vi "Seq Station Part Config.vi"(6 "User Name":string="Jon", 8 "Level":i32, 10 "station default states":T1[](array[typedef]) {"LIN INFO"."NAD" format="%.0x"; "LIN INFO"."ADCS LIN"."HW select" items=["NI-XNET", "NI-CAN"]; "LVDT Status"."LVDT's stored config"."Lower Limit" format="%.2f"; "LVDT Status"."LVDT's stored config"."Upper Limit" format="%.2f"; "Store Data"."Sun Shade Open Force Limits"."Variance" format="%.2g"; "Store Data"."Sun Shade Open Force Limits"."Truncation End" format="%.2g"; "Store Data"."Sun Shade Open Force Limits"."Truncation Start" format="%.2g"; "Store Data"."Sun Shade Open Force Limits"."Avg Max" format="%.2g"; "Store Data"."Sun Shade Open Force Limits"."Avg Min" format="%.2g"; "Store Data"."Sun Shade Open Force Limits"."Overall Max" format="%.2g"; "Store Data"."Sun Shade Open Force Limits"."Overall Min" format="%.2g"; "Store Data"."Sun Shade Close Force Limits"."Variance" format="%.2g"; "Store Data"."Sun Shade Close Force Limits"."Truncation End" format="%.2g"; "Store Data"."Sun Shade Close Force Limits"."Truncation Start" format="%.2g"; "Store Data"."Sun Shade Close Force Limits"."Avg Max" format="%.2g"; "Store Data"."Sun Shade Close Force Limits"."Avg Min" format="%.2g"; "Store Data"."Sun Shade Close Force Limits"."Overall Max" format="%.2g"; "Store Data"."Sun Shade Close Force Limits"."Overall Min" format="%.2g"; "Store Data"."Motion Data Array"."Motion Data Limits"."LIN Msg"."Msg" format="%02x"; "Store Data"."Motion Data Array"."Motion Data Limits"."LIN Msg"."ID" format="%02x"}, 11 "Base Path":path=path "C:/Labview Code") -> ()   [LabVIEW 2018]
uses:
  02.Type Def's/main state cluster.ctl
  02.Type Def's/All Switch Configuration Cluster.ctl
  02.Type Def's/All Motions.ctl
  02.Type Def's/EOL Switch Value Configuration Cluster.ctl
  02.Type Def's/EOL Switch Max Min Check Cluster.ctl
  02.Type Def's/station nvh config.ctl
  02.Type Def's/station rs232 port map.ctl
  02.Type Def's/station ethernet address map.ctl
  02.Type Def's/station paths.ctl
  02.Type Def's/EOL Save Module Test Data Control.ctl
  02.Type Def's/EOL Motion Database Table.ctl
  05.UserVI's/type defs/17x Audit Motion Data Seq Control.ctl
  05.UserVI's/type defs/17x AP Data Type.ctl
  05.UserVI's/type defs/17x Sunshade Limts Seq.ctl
  02.Type Def's/EOL Module Info Control.ctl
  02.Type Def's/station DI map.ctl
  05.UserVI's/type defs/EOL Global Digital Input Control.ctl
  02.Type Def's/control refs.ctl
  02.Type Def's/station motion data indicator.ctl
  02.Type Def's/Screen Motion Data.ctl
  02.Type Def's/Pass Fail Control.ctl
  02.Type Def's/station hmi.ctl
  02.Type Def's/lvdt name val pair.ctl
  02.Type Def's/individual station status.ctl
  02.Type Def's/misc station config.ctl
  05.UserVI's/Lambda Power/power supply types.ctl
  05.UserVI's/type defs/EOL LVDT's Check Controller.ctl
  05.UserVI's/LVDT's/lvdt precision.ctl
  02.Type Def's/sequence state.ctl
  05.UserVI's/sequence/type defs/Sequence Info.ctl
  05.UserVI's/type defs/EOL Part Setup.ctl
  02.Type Def's/All Communication Types.ctl
  05.UserVI's/type defs/Communication with Motors.ctl
  05.UserVI's/type defs/RAP Signal Control.ctl
  05.UserVI's/type defs/EOL Motor Type.ctl
  02.Type Def's/station LIN config.ctl
  03.Inalfa LIN/LIN Device.ctl
  <vilib>/CMC.AME/Inalfa ADCS/Ctl'Def/ADCS_LIN info.ctl
  C:/Program Files (x86)/National Instruments/LabVIEW 2018/vi.lib/CMC.AME/Inalfa TS LIN/TOSUN/TSMaster/bin/Interop.TSMasterAPI.dll
  Program Files (x86)/National Instruments/LabVIEW 2018/vi.lib/CMC.AME/Inalfa TS LIN/TOSUN/TSMaster/bin/Interop.TSMasterAPI.dll
  06.Test Loop/Sub'VIs/Type Def's/Config Info.ctl
panel:
  in  "LIN Msg Editor":bool
  in  "st4":bool
  in  "st3":bool
  in  "shade config":bool
  in  "st0":bool
  in  "Part Type":u16(ring) items=["OE", "EX1H", "EX1E"]
  in  "st1":bool
  in  "Exit":bool
  in  "st2":bool
  # "Part Configuration"
  # "Sunroof Barcode"
  # "Pallet Number"
  # "Part Type"
  # "Application Status"
  # "Current Step"
  # "Cycle Time"
  # "Pass / Fail"
  # "Shade Close"
  # "Actual Data"
  # "Limits"
  # "Avg Current"
  # "Run Time"
  # "Speed"
  # "Noise Test"
  # "Position"
  # "Shade Open"
  # "Actual Data"
  # "Limits"
  # "Avg Current"
  # "Run Time"
  # "Speed"
  # "Noise Test"
  # "Position"
  # "Vent Close"
  # "Actual Data"
  # "Limits"
  # "Avg Current"
  # "Run Time"
  # "Speed"
  # "Noise Test"
  # "Position"
  # "Vent Open"
  # "Actual Data"
  # "Limits"
  # "Avg Current"
  # "Run Time"
  # "Speed"
  # "Noise Test"
  # "Position"
  # "Slide Close"
  # "Actual Data"
  # "Limits"
  # "Avg Current"
  # "Run Time"
  # "Speed"
  # "Noise Test"
  # "Position"
  # "Slide Open"
  # "Actual Data"
  # "Limits"
  # "Avg Current"
  # "Run Time"
  # "Speed"
  # "Noise Test"
  # "Position"
  # "Min"
  # "N"
  # "Min"
  # "Start"
  # "N"
  # "Max"
  # "N"
  # "Max"
  # "N"
  # "End"
  # "Min"
  # "N"
  # "Min"
  # "Start"
  # "N"
  # "Max"
  # "N"
  # "Max"
  # "N"
  # "End"
  # "Min"
  # "Max"
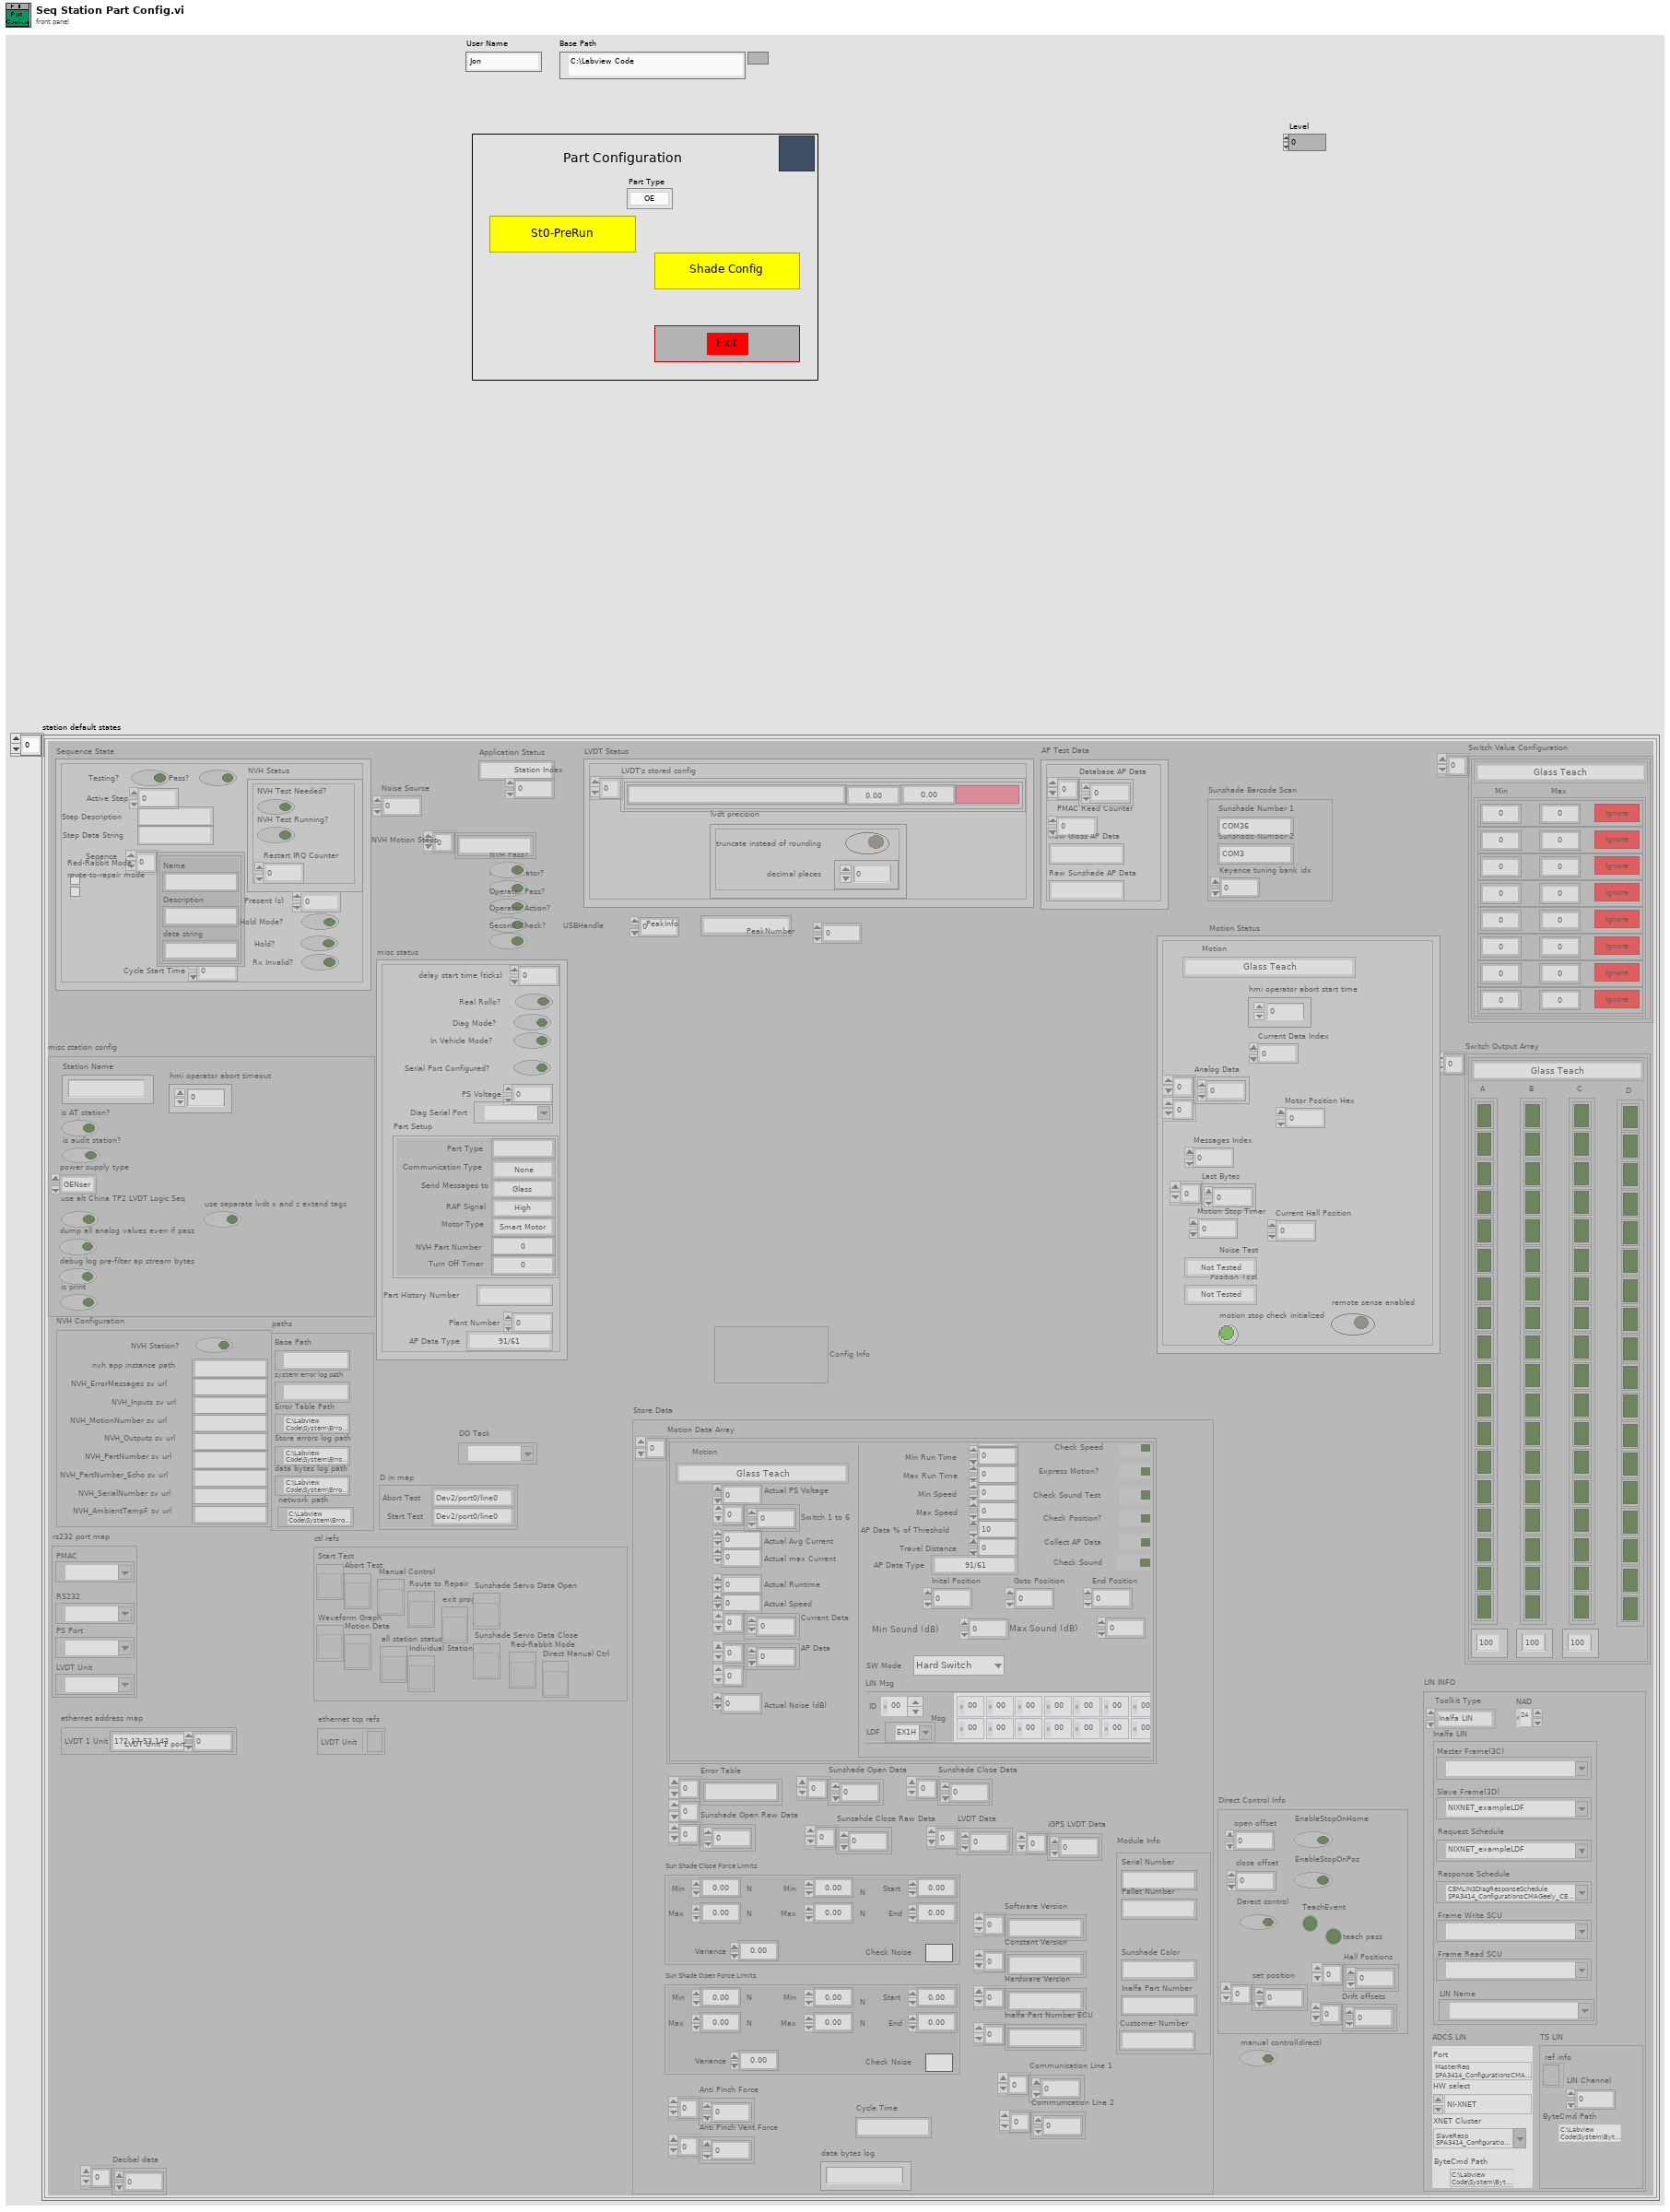
[diagram p1: front panel]
types:
  T1 = typedef "main state cluster.ctl" = cluster{"Application Status":string, "Switch Output Array":T2[], "Switch Value Configuration":T4[], "NVH Configuration":T6, "rs232 port map":T7, "ethernet address map":T8, "paths":T9, "Station Index":i32, "Store Data":T10, "D in map":T16, "DO Task":refnum<k21>, "ctl refs":T18, "misc station config":T19, "ethernet tcp refs":cluster{"LVDT Unit":refnum<k5>}, "Sunshade Barcode Scan":cluster{"Sunshade Number 2":string, "Sunshade Number 1":string, "Keyence tuning bank idx":i32}, "AP Test Data":cluster{"Raw Sunshade AP Data":string, "Raw Glass AP Data":string, "PMAC Read Counter":dbl, "Database AP Data":dbl[]}, "Motion Status":cluster{"hmi operator abort start time":u32, "Current Data Index":i32, "Analog Data":sgl[][], "Motor Position Hex":u16, "Messages Index":u16, "Last Bytes":u8[], "Current Hall Position":i16, "Motion Stop Timer":u32, "Position Test":T21, "Noise Test":T21, "motion stop check initialized":bool, "remote sense enabled":bool, "Motion":T3}, "LVDT Status":cluster{"LVDT's stored config":T22[], "lvdt precision":T23}, "Sequence State":T24, "misc status":cluster{"delay start time (ticks)":u32, "In Vehicle Mode?":bool, "Diag Mode?":bool, "Serial Port Configured?":bool, "PS Voltage":dbl, "Diag Serial Port":refnum<visa-resource-name>, "Part Setup":T26, "Part History Number":string, "Plant Number":u8, "AP Data Type":T13, "Real Rollo?":bool}, "NVH Operator?":bool, "NVH Pass?":bool, "Operator Pass?":bool, "Operator Action?":bool, "Noise Source":u32, "USBHandle":i32, "PeakInfo":string, "PeakNumber":i32, "NVH Motion Steps":string[], "Second Check?":bool, "Decibel data":dbl[], "Direct Control Info":cluster{"EnableStopOnHome":bool, "EnableStopOnPos":bool, "TeachEvent":bool, "open offset":i32, "close offset":i32, "Derect control":bool, "set position":i32[], "teach pass ":bool, "Drift offsets":i32[], "Hall Positions":i32[]}, "manual control(direct)":bool, "LIN INFO":T31, "Config Info":T34}
  T2 = typedef "All Switch Configuration Cluster.ctl" = cluster{"All Motions":T3, "A":bool[], "B":bool[], "C":bool[], "D":bool[], "A activation time (ms)":u32, "B activation time (ms)":u32, "C activation time (ms)":u32}
  T3 = typedef "All Motions.ctl" = enum16{"Glass Teach", "Glass Slide Open", "Glass Slide Close", "Glass Vent Open", "Glass Vent Close", "Sunshade Teach", "Sunshade Open", "Sunshade Close", "Idle", "Sunshade Open 2", "Sunshade Close 2", "Glass Slide Open Sunshade Open", "Glass Slide Open Sunshade Close", "Glass Slide Close Sunshade Open", "Glass Slide Close Sunshade Close", "Glass Vent Open Sunshade Open", "Glass Vent Open Sunshade Close", "Glass Vent Close Sunshade Open", "Glass Vent Close Sunshade Close", "Express Glass Slide Open", "Express Glass Slide Close", "Express Glass Vent Open", "Express Glass Vent Close", "Express Sunshade Open", "Express Sunshade Close", "Express Sunshade Open 2", "Express Sunshade Close 2", "Express Glass Slide Open Sunshade Open", "Express Glass Slide Open Sunshade Close", "Express Glass Slide Close Sunshade Open", "Express Glass Slide Close Sunshade Close", "Express Glass Vent Open Sunshade Open", "Express Glass Vent Open Sunshade Close", "Express Glass Vent Close Sunshade Open", "Express Glass Vent Close Sunshade Close", "Goto Position Glass", "Goto Position Sunshade", "Sunshade Teach 2"}
  T4 = typedef "EOL Switch Value Configuration Cluster.ctl" = cluster{"All Motions":T3, "Array":T5[]}
  T5 = typedef "EOL Switch Max Min Check Cluster.ctl" = cluster{"Min":dbl, "Max":dbl, "Check?":bool}
  T6 = typedef "station nvh config.ctl" = cluster{"NVH Station?":bool, "nvh app instance path":string, "NVH_ErrorMessages sv url":string, "NVH_Inputs sv url":string, "NVH_MotionNumber sv url":string, "NVH_Outputs sv url":string, "NVH_PartNumber sv url":string, "NVH_PartNumber_Echo sv url":string, "NVH_SerialNumber sv url":string, "NVH_AmbientTempF sv url":string}
  T7 = typedef "station rs232 port map.ctl" = cluster{"PMAC":refnum<visa-resource-name>, "PS Port":refnum<visa-resource-name>, "LVDT Unit":refnum<visa-resource-name>, "RS232":refnum<visa-resource-name>}
  T8 = typedef "station ethernet address map.ctl" = cluster{"LVDT 1 Unit":string, "LVDT Unit 1 port":u16}
  T9 = typedef "station paths.ctl" = cluster{"Base Path":path, "system error log path":path, "Error Table Path":path, "Store errors log path":path, "data bytes log path":path, "network path":path}
  T10 = typedef "EOL Save Module Test Data Control.ctl" = cluster{"Motion Data Array":T11[], "Error Table":string[][], "Sun Shade Close Force Limits":T14, "Sun Shade Open Force Limits":T14, "Sunshade Open Data":sgl[], "Sunshade Close Data":sgl[], "Module Info":T15, "Sunsahde Close Raw Data":sgl[], "Sunshade Open Raw Data":sgl[], "Software Version":string[], "Constant Version":string[], "Hardware Version":string[], "Inalfa Part Number ECU":string[], "LVDT Data":sgl[], "Communication Line 1":sgl[], "Communication Line 2":sgl[], "Anti Pinch Force":sgl[], "Cycle Time":string, "Anti Pinch Vent Force":sgl[], "iGPS LVDT Data":sgl[], "data bytes log":string}
  T11 = typedef "EOL Motion Database Table.ctl" = cluster{"Motion":T3, "Actual Avg Current":dbl, "Actual Runtime":dbl, "Actual Speed":dbl, "Current Data":sgl[], "Motion Data Limits":T12, "Switch 1 to 6":dbl[], "Actual PS Voltage":dbl, "AP Data":i16[][], "Actual max Current":dbl, "Actual Noise (dB)":dbl}
  T12 = typedef "17x Audit Motion Data Seq Control.ctl" = cluster{"Power Supply Voltage":dbl, "Min Avg Current":dbl, "Max Avg Current":dbl, "Min Run Time":dbl, "Max Run Time":dbl, "Min Speed":dbl, "Max Speed":dbl, "AP Data % of Threshold":dbl, "Travel Distance":dbl, "AP Data Type":T13, "Check Current":bool, "Check Run Time":bool, "Check Speed":bool, "Express Motion?":bool, "Check Sound Test":bool, "Check Position?":bool, "Collect AP Data":bool, "Inital Position":u16, "End Position":u16, "Goto Posiition":u16, "Max max Current":dbl, "Min max Current":dbl, "Check max Current":bool, "Check Sound":bool, "Min Sound (dB)":dbl, "Max Sound (dB)":dbl, "SW Mode":enum16{"Hard Switch", "Uncond Frame"}, "LIN Msg":cluster{"ID":u8, "Msg":u8[][], "LDF":refnum<k21>}}
  T13 = typedef "17x AP Data Type.ctl" = enum16{"91/61", "92/62", "93/63", "67", "68", "6F", "71", "91 Msg", "92 Msg", "93 Msg", "94 Msg", "HiRain 91", "HiRain 92 Speed", "HiRain 92 HS", "HiRain 92", "HiRain 93", "SnT"}
  T14 = typedef "17x Sunshade Limts Seq.ctl" = cluster{"Overall Min":dbl, "Overall Max":dbl, "Avg Min":dbl, "Avg Max":dbl, "Truncation Start":dbl, "Truncation End":dbl, "Variance":dbl, "Check Noise":bool}
  T15 = typedef "EOL Module Info Control.ctl" = cluster{"Serial Number":string, "Pallet Number":string, "Sunshade Color":string, "Inalfa Part Number":string, "Customer Number":string}
  T16 = typedef "station DI map.ctl" = cluster{"Abort Test":T17, "Start Test":T17}
  T17 = typedef "EOL Global Digital Input Control.ctl" = enum16{"Dev2/port0/line0", "Dev2/port0/line1", "Dev2/port0/line2", "Dev2/port0/line3", "Dev2/port0/line4", "Dev2/port0/line5", "Dev2/port0/line6", "Dev2/port0/line7", "Dev2/port1/line0", "Dev2/port1/line1", "Dev2/port1/line2", "Dev2/port1/line3", "Dev2/port1/line4", "Dev2/port1/line5", "Dev2/port1/line6", "Dev2/port1/line7", "Dev2/port2/line0", "Dev2/port2/line1", "Dev2/port2/line2", "Dev2/port2/line3", "Dev2/port2/line4", "Dev2/port2/line5", "Dev2/port2/line6", "Dev2/port2/line7", "Prerun Start Test", "Prerun Abort Test", "Audit Start Test", "Audit Abort Test", "Dev2/port3/line4", "Dev2/port3/line5", "Breakin Start Test", "Breakin Abort Test", "Not Implemented"}
  T18 = typedef "control refs.ctl" = cluster{"Start Test":refnum<vi>, "Abort Test":refnum<vi>, "Manual Control":refnum<vi>, "Route to Repair":refnum<vi>, "Waveform Graph":refnum<vi>, "Motion Data":refnum<vi>, "all station status":refnum<vi>, "Individual Station Status":refnum<vi>, "exit program":refnum<vi>, "Sunshade Servo Data Open":refnum<vi>, "Sunshade Servo Data Close":refnum<vi>, "Red-Rabbit Mode":refnum<vi>, "Direct Manual Ctrl":refnum<vi>}
  T19 = typedef "misc station config.ctl" = cluster{"Station Name":string, "is AT station?":bool, "is audit station?":bool, "power supply type":T20, "use alt China TP2 LVDT Logic Seq":bool, "hmi operator abort timeout":u32, "dump all analog values even if pass":bool, "debug log pre-filter ap stream bytes":bool, "use separate lvdt x and z extend tags":bool, "is print":bool}
  T20 = typedef "power supply types.ctl" = enum16{"GENser", "ZUPser", "GENeth", "Manual", "ITECH"}
  T21 = typedef "Pass Fail Control.ctl" = enum16{"Not Tested", "Pass", "Fail"}
  T22 = typedef "EOL LVDT's Check Controller.ctl" = cluster{"Upper Limit":dbl, "Lower Limit":dbl, "LVDT Name":string, "Check":bool}
  T23 = typedef "lvdt precision.ctl" = cluster{"truncate instead of rounding":bool, "decimal places":u8}
  T24 = typedef "sequence state.ctl" = cluster{"Step Description":string, "Cycle Start Time":u32, "Step Data String":string, "Pass?":bool, "Seqence":T25[], "Active Step":u8, "Testing?":bool, "Red-Rabbit Mode":bool, "route-to-repair mode":bool, "NVH Status":cluster{"Restart IRQ Counter":u8, "NVH Test Needed?":bool, "NVH Test Running?":bool}, "Present (s)":dbl, "Hold Mode?":bool, "Hold?":bool, "Rx Invalid?":bool}
  T25 = typedef "Sequence Info.ctl" = cluster{"Name":string, "Description":string, "data string":string}
  T26 = typedef "EOL Part Setup.ctl" = cluster{"Communication Type":T27, "Send Messages to":T28, "RAP Signal":T29, "Motor Type":T30, "NVH Part Number":u16, "Turn Off Timer":u16, "Part Type":string}
  T27 = typedef "All Communication Types.ctl" = enum16{"None", "CAN", "RS 232", "RS 232 LIN", "GM LIN", "SnT LIN", "K Line", "Robel CAN", "P42M-Continental", "Inalfa SCU LIN", "Spare 3"}
  T28 = typedef "Communication with Motors.ctl" = enum16{"Glass", "Rollo", "Both"}
  T29 = typedef "RAP Signal Control.ctl" = enum16{"High", "Low", "None"}
  T30 = typedef "EOL Motor Type.ctl" = enum16{"Smart Motor", "Sensor Motor"}
  T31 = typedef "station LIN config.ctl" = cluster{"Toolkit Type":enum16{"Inalfa LIN", "ADCS LIN", "TS LIN"}, "NAD":u8, "Inalfa LIN":T32, "ADCS LIN":T33, "TS LIN":cluster{"ref info":refnum<k24>, "LIN Channel":i32, "ByteCmd Path":path}}
  T32 = typedef "LIN Device.ctl" = cluster{"Master Frame(3C)":refnum<k21>, "Slave Frame(3D)":refnum<k21>, "Request Schedule":refnum<k21>, "Response Schedule":refnum<k21>, "Frame Write SCU":refnum<k21>, "Frame Read SCU":refnum<k21>, "LIN Name":refnum<k21>}
  T33 = typedef "ADCS_LIN info.ctl" = cluster{"Port":string, "HW select":u16, "XNET Cluster":string, "ByteCmd Path":path}
  T34 = typedef "Config Info.ctl" = variant
  T35 = cluster{"Base Path":path, "Station Name":string, "Error":errorcluster, "station default states":T1[]}
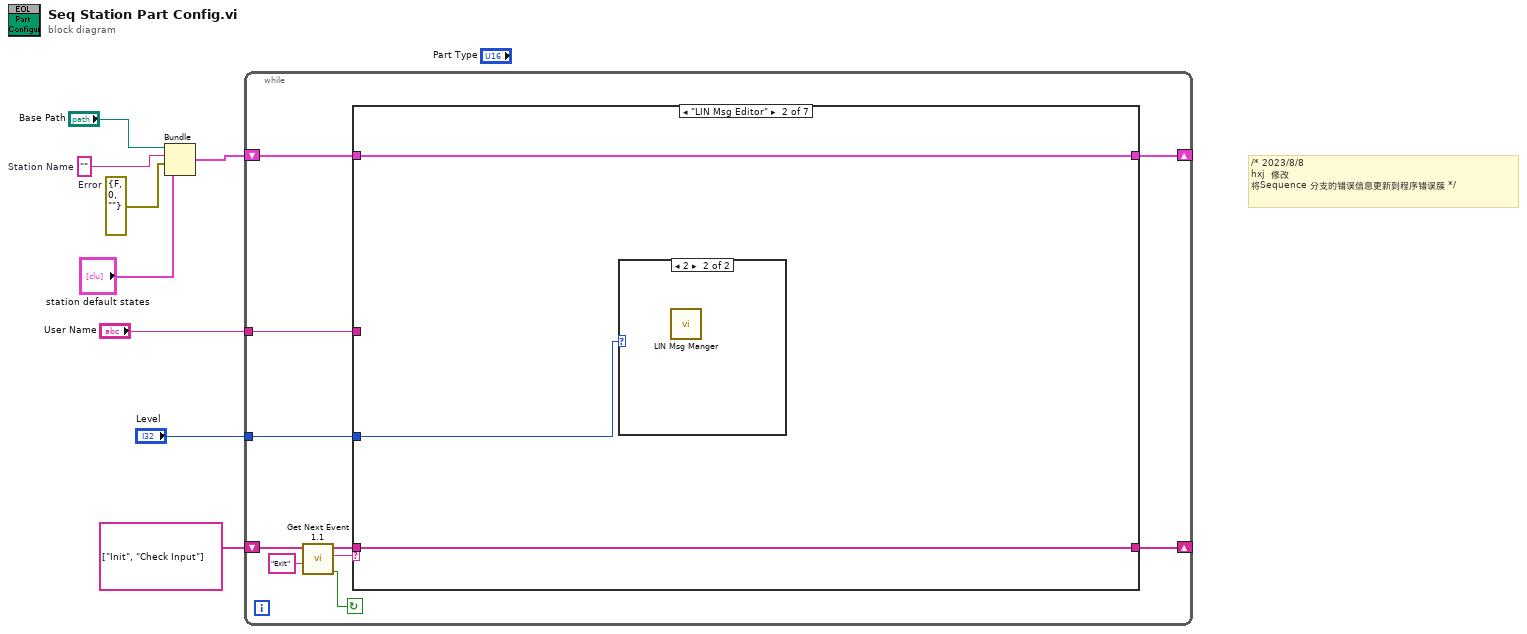
[diagram p0: block diagram]
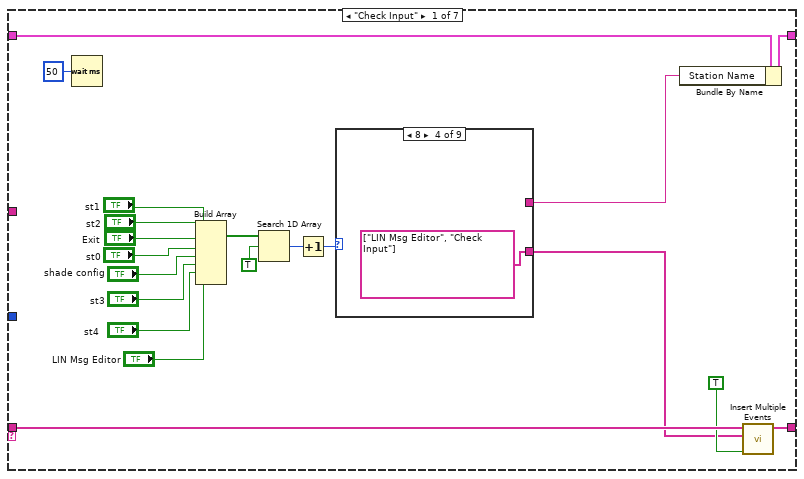
[diagram p2: hidden frame]
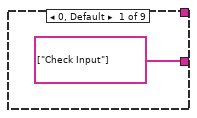
[diagram p3: hidden frame]
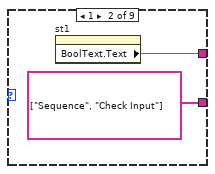
[diagram p4: hidden frame]
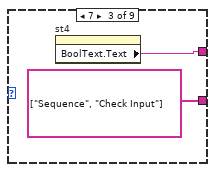
[diagram p5: hidden frame]
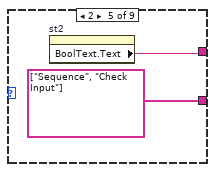
[diagram p6: hidden frame]
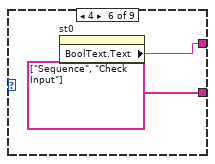
[diagram p7: hidden frame]
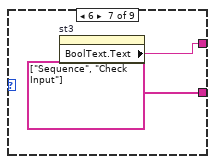
[diagram p8: hidden frame]
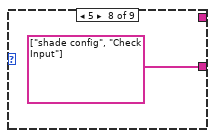
[diagram p9: hidden frame]
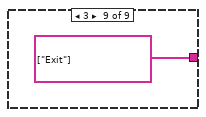
[diagram p10: hidden frame]
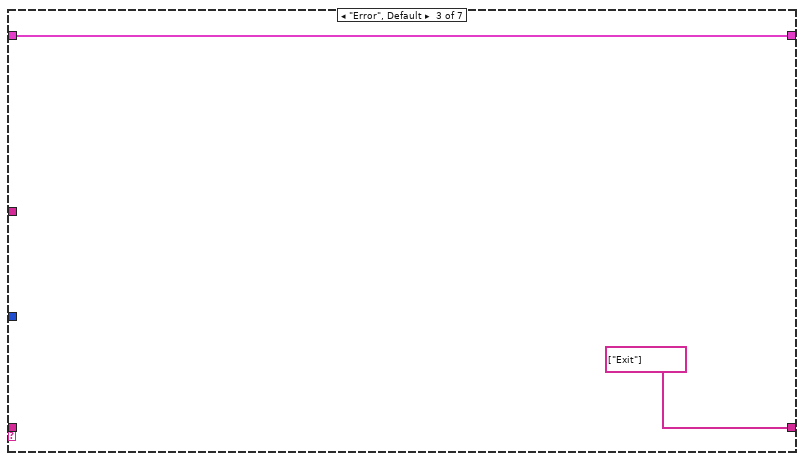
[diagram p12: hidden frame]
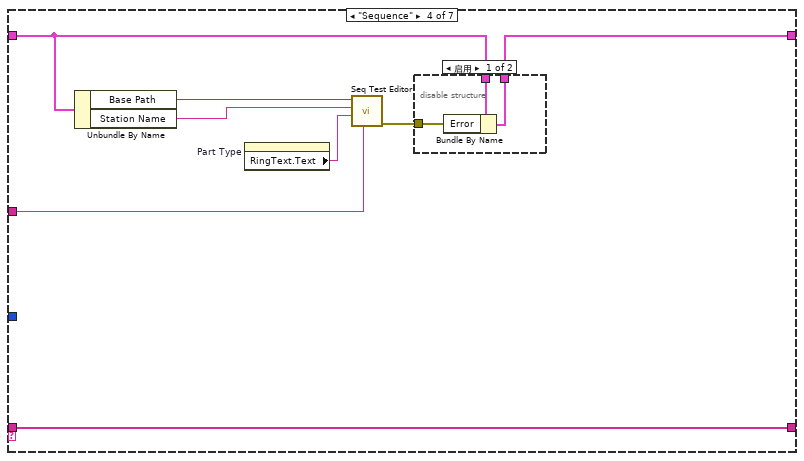
[diagram p13: hidden frame]
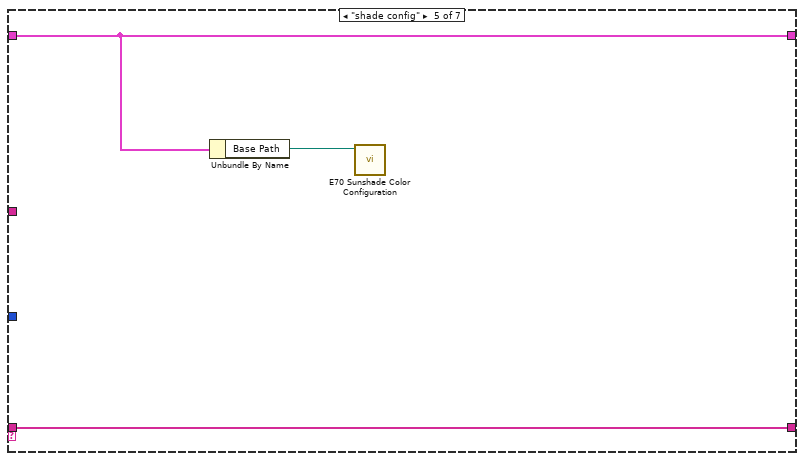
[diagram p15: hidden frame]
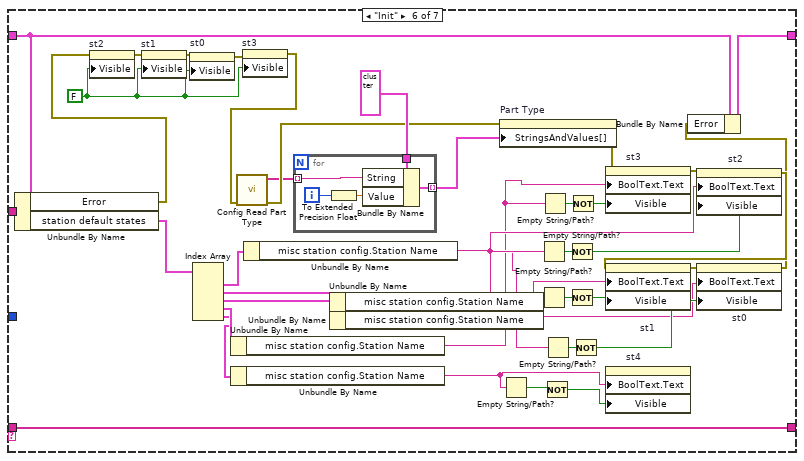
[diagram p16: hidden frame]
diagram:
  w4 = errorcluster {"status"=FALSE, "code"=0, "source"=""}  # Error
  w5 = ""  # Station Name
  # "/* 2023/8/8\nhxj  修改\n将Sequence 分支的错误信息更新到程序错误簇 */"
  n1 = Bundle("Base Path"="Base Path", "Station Name"=w5, "Error"=w4, "station default states"="station default states") -> (w7:T35)  [unwired: 1 in]
  n2 = while {
    shift-right: [w16] -> _
    shift-left: string[] ["Init", "Check Input"] -> [w15]
    shift-right: [w11] -> _
    shift-left: w7 -> [w12]
    tunnel: "User Name" -> [w10]
    tunnel: "Level" -> [w9]
    stop <- w14 continue-if-true
    n3 = call "Get Next Event 1.1.vi"("Exit Event"="Exit", "event queue in"=w15) -> ("Condition (Exit:F)"=w14:bool, "next event"=w13:string, "event queue out"=w17:string[])  [unwired: 6 in, 1 out]
    n4 = case shown="\"LIN Msg Editor\"" w13 {
      tunnel: w17 -> [w37 w54 _ w65 w70 w111 w118]
      tunnel: [w38 w54 string[] ["Exit"] ("event queue out") w65 w70 w111 w118] -> w16
      tunnel: w12 -> [w35 w55 w57 w60 w71 w107 w117]
      tunnel: [w34 w55 w57 w58 w71 w106 w117] -> w11
      tunnel: w10 -> [_ _ _ w61 _ _ _]
      tunnel: w9 -> [_ w53 _ _ _ _ _]
      frame "Check Input" {
        n5 = Wait (ms)(milliseconds to wait=u32 50) -> ()  [unwired: 1 out]
        n6 = Build Array("st1", "st2", "Exit", "st0", "shade config", "st3", "st4", "LIN Msg Editor") -> (w32:bool[])
        n7 = Search 1D Array(1D array=w32, element=TRUE) -> (index of element=w28:i32)  [unwired: 1 in]
        n8 = Increment(x=w28) -> (x+1=w27:i32)
        n9 = case shown="8" w27 {
          tunnel: [string[] ["Check Input"] string[] ["Sequence", "Check Input"] string[] ["Sequence", "Check Input"] string[] ["LIN Msg Editor", "Check Input"] string[] ["Sequence", "Check Input"] string[] ["Sequence", "Check Input"] string[] ["Sequence", "Check Input"] string[] ["shade config", "Check Input"] string[] ["Exit"]] -> w26
          tunnel: [_ w40 w42 _ w45 w47 w49 _ _] -> w24
          frame 0, Default {
          }
          frame 1 {
            n10 = property on="st1" class="Bool"() -> ("BoolText.Text"=w40:string)  [unwired: 2 in, 2 out]
          }
          frame 7 {
            n11 = property on="st4" class="Bool"() -> ("BoolText.Text"=w42:string)  [unwired: 2 in, 2 out]
          }
          frame 8 {
          }
          frame 2 {
            n12 = property on="st2" class="Bool"() -> ("BoolText.Text"=w45:string)  [unwired: 2 in, 2 out]
          }
          frame 4 {
            n13 = property on="st0" class="Bool"() -> ("BoolText.Text"=w47:string)  [unwired: 2 in, 2 out]
          }
          frame 6 {
            n14 = property on="st3" class="Bool"() -> ("BoolText.Text"=w49:string)  [unwired: 2 in, 2 out]
          }
          frame 5 {
          }
          frame 3 {
          }
        }
        n15 = Bundle By Name(cluster=w35, "Station Name"=w24) -> (w34:T35)
        n16 = call "Insert Multiple Events.vi"("Insert all? (T)"=TRUE, "Events to Insert"=w26, "Event queue in"=w37) -> ("Event queue out"=w38:string[])  [unwired: 4 in]
      }
      frame "LIN Msg Editor" {
        n17 = case shown="2" w53 {
          frame 0, Default {
          }
          frame 2 {
            n18 = call <vilib>:"LIN Msg Manger.vi"() -> ()  [unwired: 12 in]
          }
        }
      }
      frame "Error", Default {
      }
      frame "Sequence" {
        n19 = Unbundle By Name(w60) -> ("Base Path"=w64:path, "Station Name"=w62:string)
        n20 = property on="Part Type" class="Ring (严格)"() -> ("RingText.Text"=w63:string)  [unwired: 2 in, 2 out]
        n21 = call "Seq Test Editor.vi"("User Name"=w61, "Part Type"=w63, "Station"=w62, "Base Path"=w64) -> ("Sys Error Out"=w59:errorcluster)  [unwired: 7 in]
        n22 = disable-structure shown="启用" {
          disable-tunnel: w60 -> [w68 w69]
          disable-tunnel: w59 -> [w67 _]
          disable-tunnel: [w66 w69] -> w58
          frame Enabled {
            n23 = Bundle By Name(cluster=w68, "Error"=w67) -> (w66:T35)
          }
          frame Disabled {
          }
        }
      }
      frame "shade config" {
        n24 = Unbundle By Name(w71) -> ("Base Path"=w72:path)
        n25 = call "E70 Sunshade Color Configuration.vi"("Base Path"=w72) -> ()  [unwired: 11 in]
      }
      frame "Init" {
        w89 = FALSE ("Visible")
        n26 = Unbundle By Name(w107) -> ("Error"=w88:errorcluster, "station default states"=w93:T1[])
        n27 = property on="st2" class="Bool"(error in=w88, "Visible"=w89) -> (error out=w95:errorcluster)  [unwired: 1 in, 1 out]
        n28 = property on="st1" class="Bool"(error in=w95, "Visible"=w89) -> (error out=w94:errorcluster)  [unwired: 1 in, 1 out]
        n29 = property on="st0" class="Bool"(error in=w94, "Visible"=w89) -> (error out=w87:errorcluster)  [unwired: 1 in, 1 out]
        n30 = Index Array(array=w93) -> (element #1=w104:T1, element #2=w103:T1, element #3=w102:T1, element #4=w83:T1, element #5=w76:T1)  [unwired: 5 in]
        n31 = Unbundle By Name(w83) -> ("misc station config.Station Name"=w80:string)
        n32 = Unbundle By Name(w76) -> ("misc station config.Station Name"=w73:string)
        n33 = property on="st3" class="Bool"(error in=w87, "Visible"=w89) -> (error out=w86:errorcluster)  [unwired: 1 in, 1 out]
        n34 = call "Config Read Part Type.vi"("Error In"=w86) -> ("Error Out"=w108:errorcluster, "Part Types"=w105:string[])  [unwired: 8 in, 1 out]
        n35 = Unbundle By Name(w104) -> ("misc station config.Station Name"=w77:string)
        n36 = for {
          tunnel: cluster{"String":string, "Value":ext} {"String"="", "Value"=0.0} -> [w116]
          tunnel: w105 -> [w114] mode=indexing
          tunnel: [w113] -> w110 mode=indexing
          i -> [w112]
          n37 = To Extended Precision Float(1:w112) -> (0:w115:ext)
          n38 = Bundle By Name(cluster=w116, "String"=w114, "Value"=w115) -> (w113:cluster{"String":string, "Value":ext})
        }
        n39 = Unbundle By Name(w103) -> ("misc station config.Station Name"=w82:string)
        n40 = Unbundle By Name(w102) -> ("misc station config.Station Name"=w81:string)
        n41 = property on="Part Type" class="Ring (严格)"(error in=w108, "StringsAndValues[]"=w110) -> (error out=w79:errorcluster)  [unwired: 1 in, 1 out]
        n42 = Empty String/Path?(string/path=w73) -> (empty?=w75:bool)
        n43 = Empty String/Path?(string/path=w81) -> (empty?=w101:bool)
        n44 = Empty String/Path?(string/path=w82) -> (empty?=w99:bool)
        n45 = Empty String/Path?(string/path=w80) -> (empty?=w84:bool)
        n46 = Not(x=w75) -> (.not. x?=w74:bool)
        n47 = Empty String/Path?(string/path=w77) -> (empty?=w98:bool)
        n48 = Not(x=w101) -> (.not. x?=w100:bool)
        n49 = Not(x=w99) -> (.not. x?=w97:bool)
        n50 = Not(x=w84) -> (.not. x?=w85:bool)
        n51 = Not(x=w98) -> (.not. x?=w96:bool)
        n52 = property on="st3" class="Bool"(error in=w79, "BoolText.Text"=w80, "Visible"=w85) -> (error out=w78:errorcluster)  [unwired: 1 in, 1 out]
        n53 = property on="st4" class="Bool"("BoolText.Text"=w73, "Visible"=w74) -> ()  [unwired: 2 in, 2 out]
        n54 = property on="st2" class="Bool"(error in=w78, "BoolText.Text"=w81, "Visible"=w100) -> (error out=w92:errorcluster)  [unwired: 1 in, 1 out]
        n55 = property on="st1" class="Bool"(error in=w92, "BoolText.Text"=w82, "Visible"=w97) -> (error out=w91:errorcluster)  [unwired: 1 in, 1 out]
        n56 = property on="st0" class="Bool"(error in=w91, "BoolText.Text"=w77, "Visible"=w96) -> (error out=w90:errorcluster)  [unwired: 1 in, 1 out]
        n57 = Bundle By Name(cluster=w107, "Error"=w90) -> (w106:T35)
      }
      frame "Exit" {
      }
    }
  }
